vi "Experiment Helper.vi"(0 "object in":refnum<class "Experiment.lvclass">, 5 "error in (no error)":errorcluster) -> (14 "object out":refnum<class "Experiment.lvclass">, 19 "error out":errorcluster)   [LabVIEW 2021, in "Experiment.lvclass"]
uses:
  Experiment.lvclass
panel:
  in  "Cluster":T1
  in  "Array of Levels in Syringe":dbl[](array[numeric])
  in  "element":T2
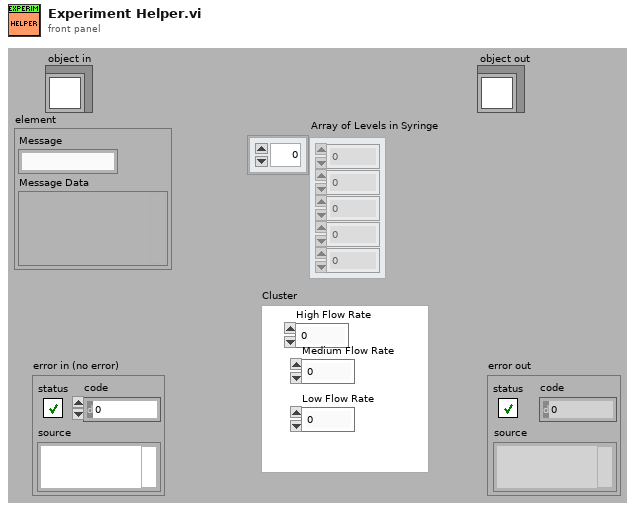
[diagram p1: front panel]
types:
  T1 = cluster{"High Flow Rate":dbl, "Medium Flow Rate":dbl, "Low Flow Rate":dbl}
  T2 = cluster{"Message":string, "Message Data":variant}
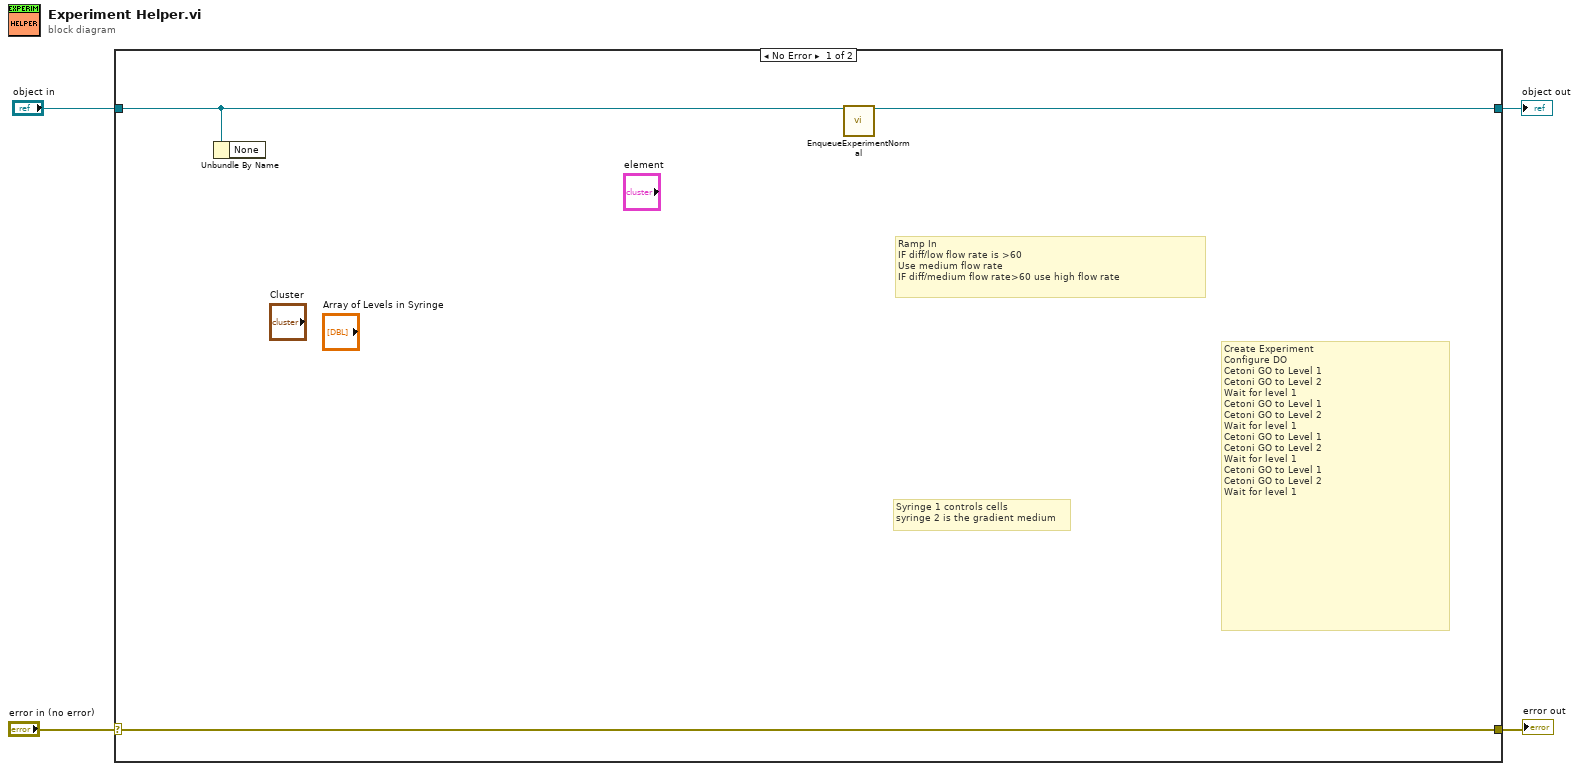
[diagram p0: block diagram]
diagram:
  n1 = case shown="No Error" "error in (no error)" {
    selector: "error in (no error)" -> [w8 w10]
    tunnel: [w8 w10] -> w3
    tunnel: [w6 w9] -> w1
    tunnel: "object in" -> [w7 w9]
    frame No Error {
      # "Ramp In\nIF diff/low flow rate is >60\nUse medium flow rate\nIF diff/medium flow rate>60 use high flow rate"
      # "Syringe 1 controls cells \nsyringe 2 is the gradient medium"
      # "Create Experiment\nConfigure DO\nCetoni GO to Level 1\nCetoni GO to Level 2\nWait for level 1\nCetoni GO to Level 1\nCetoni GO to Level 2\nWait for level 1\nCetoni GO to Level 1\nCetoni GO to Level 2\nWait for level 1\nCetoni GO to Level 1\nCetoni GO to Level 2\nWait for level 1"
      n2 = Unbundle By Name(w7) -> ()  [unwired: 1 out]
      n3 = call-dynamic "EnqueueExperimentNormal.vi"("object in"=w7) -> (2:w5, "object out"=w6:refnum<class "Experiment.lvclass">)  [unwired: 16 in, 1 out]
    }
    frame Error {
    }
  }
  "error out" <- w3
  "object out" <- w1
